vi "DAQ.Stop.vi"(8 "error in (no error)":errorcluster, 11 "Instrument.DAQ in":refnum<class "Instrument.DAQ.lvclass">) -> (0 "error out":errorcluster, 3 "Instrument.DAQ out":refnum<class "Instrument.DAQ.lvclass">)   [LabVIEW 2019, in "Instrument.DAQ.lvclass"]
uses:
  Instrument.DAQ.lvclass
  Instrument.DAQ.lvclass/Instrument.DAQ.ctl
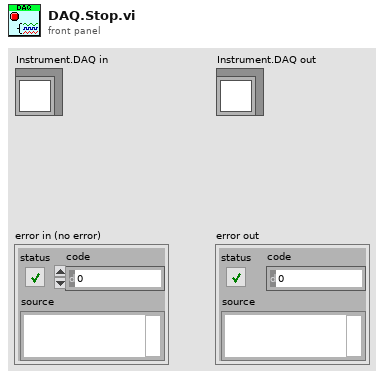
[diagram p1: front panel]
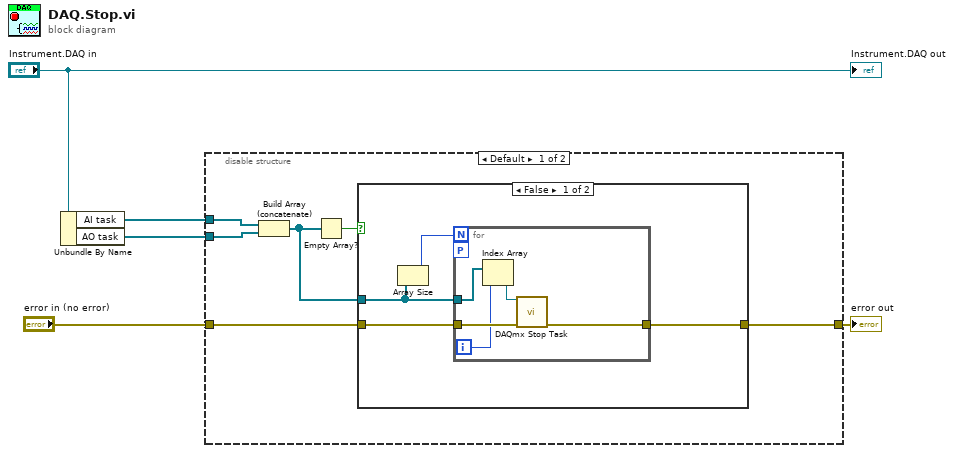
[diagram p0: block diagram]
diagram:
  n1 = Unbundle By Name("Instrument.DAQ in") -> ("AI task"=w2:refnum<k21>[], "AO task"=w3:refnum<k21>[])
  n2 = disable-structure shown="Default" {
    disable-tunnel: "error in (no error)" -> [w11 _]
    disable-tunnel: [w8 _] -> w4
    disable-tunnel: w3 -> [w9 _]
    disable-tunnel: w2 -> [w10 _]
    frame condition #0 (active) {
      n3 = Build Array (concatenate)(w10, w9) -> (w6:refnum<k21>[])
      n4 = Empty Array?(array=w6) -> (empty?=w7:bool)
      n5 = case shown="False" w7 {
        tunnel: w11 -> [w15 w21]
        tunnel: w6 -> [w13 _]
        tunnel: [w14 w21] -> w8
        frame False {
          n6 = Array Size(array=w13) -> (size(s)=w12:i32)
          n7 = for {
            N: w12 -> [_]
            tunnel: w13 -> [w18]
            tunnel: w15 -> [w20]
            tunnel: [w19] -> w14
            workers-P: _ -> [_]
            i -> [w17]
            n8 = Index Array(array=w18, index=w17) -> (element=w16:refnum<k21>)
            n9 = call <vilib>:"DAQmx Stop Task.vi"("task/channels in"=w16, "error in"=w20) -> ("error out"=w19:errorcluster)  [unwired: 12 in, 1 out]
          }
        }
        frame True {
        }
      }
    }
    frame condition #1 {
    }
  }
  "error out" <- w4
  "Instrument.DAQ out" <- "Instrument.DAQ in"
